vi "thermometer.vi"() -> (0 "temperature":dbl)   [LabVIEW 2018]
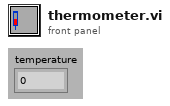
[diagram p1: front panel]
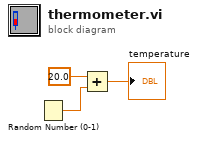
[diagram p0: block diagram]
diagram:
  n1 = Random Number (0-1)() -> (number: 0 to 1=w1:dbl)
  n2 = Add(x=20.0, y=w1) -> (x+y=→"temperature":dbl)
